vi "Harvest Selected Project Vi.vi"(0 "ActiveProject":refnum<vi>, 11 "error in":errorcluster) -> (6 "Array":refnum<vi>[](array[refnum]), 15 "error out":errorcluster)   [LabVIEW 2012, in "QuickVIew.lvlib"]
uses:
  QuickVIew.lvlib
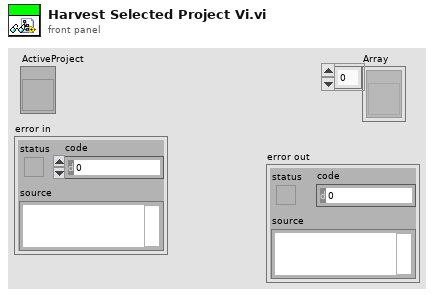
[diagram p1: front panel]
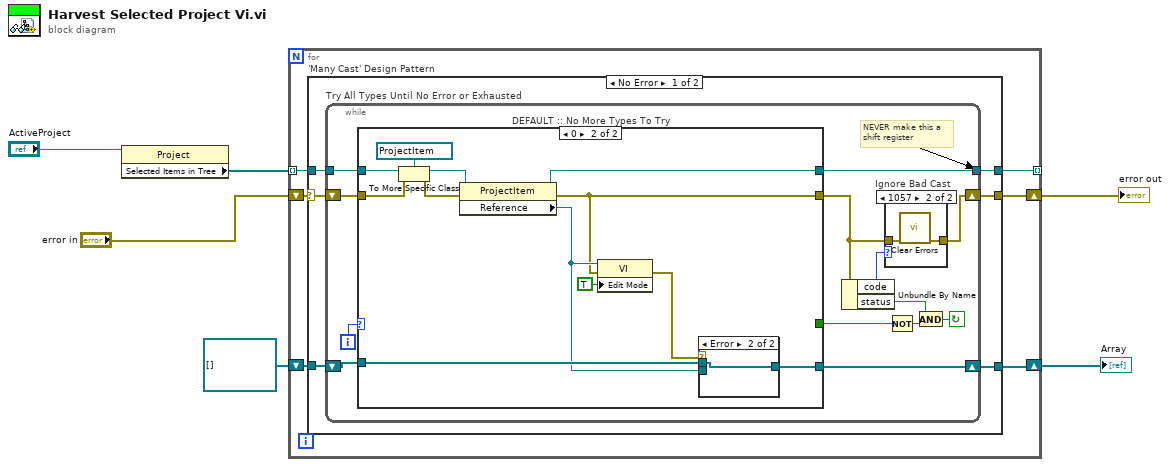
[diagram p0: block diagram]
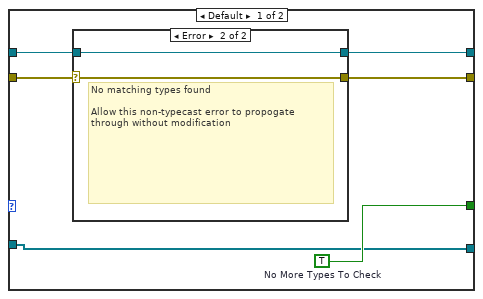
[diagram p3: hidden frame]
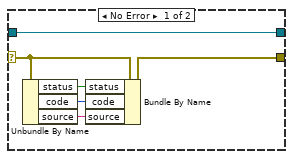
[diagram p4: hidden frame]
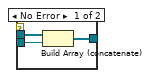
[diagram p5: hidden frame]
diagram:
  n1 = property class="Project"(reference="ActiveProject") -> ("Selected Items in Tree"=w4:refnum<vi>[])  [unwired: 1 in, 2 out]
  n2 = for {
    tunnel: w4 -> [w12] mode=indexing
    tunnel: [w10] -> _ mode=indexing
    shift-right: [w8] -> w6
    shift-left: refnum<vi>[] [] -> [w9]
    shift-right: [w7] -> w3
    shift-left: "error in" -> [w11]
    n3 = case "'Many Cast' Design Pattern" shown="No Error" w11 {
      selector: w11 -> [w15 w67]
      tunnel: w12 -> [w18 w66]
      tunnel: [w17 w66] -> w10
      tunnel: [w16 w67] -> w7
      tunnel: w9 -> [w14 w65]
      tunnel: [w13 w65] -> w8
      frame No Error {
        n4 = while "Try All Types Until No Error or Exhausted" {
          tunnel: w18 -> [w31]
          tunnel: [w30] -> w17
          shift-right: [w23] -> w16
          shift-left: w15 -> [w25]
          shift-right: [w20] -> w13
          shift-left: w14 -> [w19]
          i -> [w29]
          stop <- w28 continue-if-true
          # "NEVER make this a\nshift register"
          n5 = case "DEFAULT :: No More Types To Try" shown="0" w29 {
            tunnel: w25 -> [w37 w60]
            tunnel: w31 -> [w38 w58]
            tunnel: [w39 w49] -> w30
            tunnel: [w36 w52] -> w22
            tunnel: [w40 _] -> w27
            tunnel: [w35 w57] -> w20
            tunnel: w19 -> [w35 w56]
            frame Default {
              w40 = TRUE  # No More Types To Check
              n6 = case shown="Error" w37 {
                selector: w37 -> [w44 w47]
                tunnel: [w46 w48] -> w39
                tunnel: w38 -> [w46 w48]
                tunnel: [w45 w47] -> w36
                frame No Error {
                  n7 = Unbundle By Name(w44) -> ("status"=w43:bool, "code"=w42:i32, "source"=w41:string)
                  n8 = Bundle By Name(cluster=w44, "status"=w43, "code"=w42, "source"=w41) -> (w45:errorcluster)
                }
                frame Error {
                  # "No matching types found\n\nAllow this non-typecast error to propogate through without modification"
                }
              }
            }
            frame 0 {
              n9 = To More Specific Class(target class=refnum<vi> refnum ("Waveform Chart"), reference=w58, error in=w60) -> (specific class reference=w50:refnum<vi>, error out=w51:errorcluster)
              n10 = property class="ProjectItem"(reference=w50, error in=w51) -> (reference out=w49:refnum<vi>, error out=w52:errorcluster, "Reference"=w54:refnum<vi>)
              n11 = property class="VI"(reference=w54, error in=w52, "Edit Mode"=TRUE ("Edit Mode On Open")) -> (error out=w53:errorcluster)  [unwired: 1 out]
              n12 = case shown="Error" w53 {
                tunnel: w54 -> [w63 _]
                tunnel: [w62 w64] -> w57
                tunnel: w56 -> [w61 w64]
                frame No Error {
                  n13 = Build Array (concatenate)(w61, w63) -> (w62:refnum<vi>[])
                }
                frame Error {
                }
              }
            }
          }
          n14 = Unbundle By Name(w22) -> ("code"=w21:i32, "status"=w24:bool)
          n15 = case "Ignore Bad Cast" shown="1057" w21 {
            tunnel: [w32 w34] -> w23
            tunnel: w22 -> [w32 w33]
            frame Default {
            }
            frame 1057 {
              n16 = call <vilib>:"Clear Errors.vi"("error in (no error)"=w33) -> ("error out"=w34:errorcluster)  [unwired: 6 in]
            }
          }
          n17 = Not(x=w27) -> (.not. x?=w26:bool)
          n18 = And(x=w24, y=w26) -> (x .and. y?=w28:bool)
        }
      }
      frame Error {
      }
    }
  }
  "Array" <- w6
  "error out" <- w3
